vi "AnalogControl.vi"(0 "controller":refnum<k24>, 1 "analog input":i32, 2 "offset value":dbl, 3 "speed value":dbl, 5 "axis name":string, 7 "on/off":i32(ring) items=["Off", "On"], 9 "taskId":i32(ring) items=["TLibrary", "T01", "T02", "T03", "T04", "T05", "T06", "T07", "T08", "T09", "T10", "T11", "T12", "T13", "T14", "T15", "T16", "T17", "T18", "T19", "T20", "T21", "T22", "T23", "T24", "T25", "T26", "T27", "T28", "T29", "T30", "T31"], 11 "error in (no error)":errorcluster, 12 "scale factor":dbl=1.0, 13 "return immediately":bool) -> (4 "controller out":refnum<k24>, 15 "error out":errorcluster)   [LabVIEW 2020, in "Aerotech.lvlib"]
uses:
  Aerotech.lvlib
  C:/Users/HEP/Documents/GitHub/UCSB-Gantry-HEP/Drivers/Aerotech A3200/Bin/Aerotech.A3200.LabVIEW.dll
  UCSB-Gantry-HEP/Drivers/Aerotech A3200/Bin/Aerotech.A3200.LabVIEW.dll
  C:/Program Files (x86)/Aerotech/A3200/LabVIEW/2010/Bin/Aerotech.A3200.dll
  Program Files (x86)/Aerotech/A3200/LabVIEW/2010/Bin/Aerotech.A3200.dll
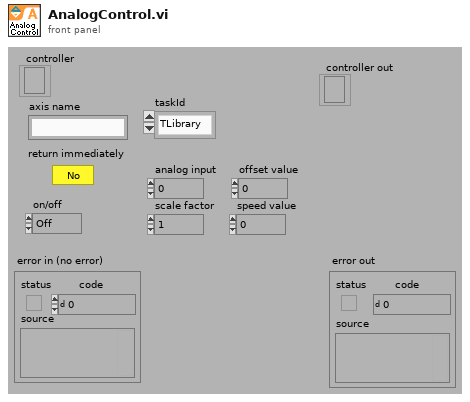
[diagram p1: front panel]
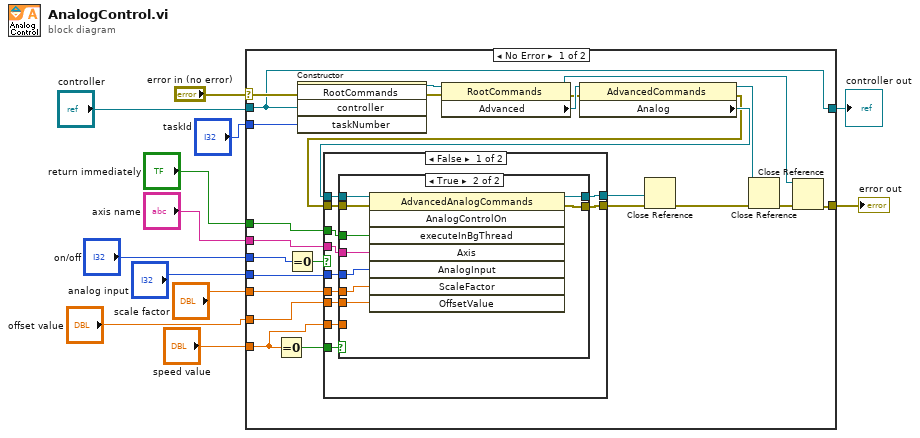
[diagram p0: block diagram]
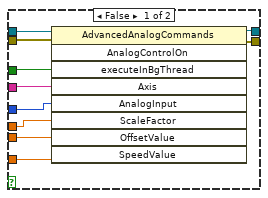
[diagram p2: hidden frame]
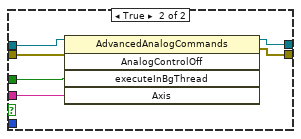
[diagram p3: hidden frame]
diagram:
  n1 = case shown="No Error" "error in (no error)" {
    selector: "error in (no error)" -> [w18 w75]
    tunnel: [w31 w75] -> w11
    tunnel: "controller" -> [w16 w74]
    tunnel: "return immediately" -> [w35 _]
    tunnel: "axis name" -> [w34 _]
    tunnel: "on/off" -> [w21 _]
    tunnel: [w16 w74] -> w1
    tunnel: "analog input" -> [w26 _]
    tunnel: "scale factor" -> [w25 _]
    tunnel: "offset value" -> [w24 _]
    tunnel: "speed value" -> [w22 _]
    tunnel: "taskId" -> [w13 _]
    frame No Error {
      n2 = Equal To 0?(x=w22) -> (x = 0?=w23:bool)
      n3 = Equal To 0?(x=w21) -> (x = 0?=w20:bool)
      n4 = constructor class="RootCommands"(error in=w18, "controller"=w16, "taskNumber"=w13) -> (reference out=w19:refnum<k24>, error out=w17:errorcluster)  [unwired: 2 in, 3 out]
      n5 = property class="RootCommands"(reference=w19, error in=w17) -> (reference out=w28:refnum<k24>, error out=w14:errorcluster, "Advanced"=w15:refnum<k24>)
      n6 = property class="AdvancedCommands"(reference=w15, error in=w14) -> (reference out=w29:refnum<k24>, error out=w36:errorcluster, "Analog"=w37:refnum<k24>)
      n7 = case shown="False" w20 {
        tunnel: w37 -> [w48 w72]
        tunnel: w36 -> [w47 w73]
        tunnel: w35 -> [w46 w71]
        tunnel: w34 -> [w45 w70]
        tunnel: [w44 w68] -> w33
        tunnel: [w43 w69] -> w32
        tunnel: w26 -> [w42 _]
        tunnel: w25 -> [w41 _]
        tunnel: w24 -> [w40 _]
        tunnel: w23 -> [w39 _]
        tunnel: w22 -> [w38 _]
        frame False {
          n8 = case shown="True" w39 {
            tunnel: w48 -> [w58 w67]
            tunnel: w47 -> [w57 w66]
            tunnel: w46 -> [w56 w65]
            tunnel: w45 -> [w55 w64]
            tunnel: [w54 w63] -> w44
            tunnel: [w53 w62] -> w43
            tunnel: w42 -> [w49 w61]
            tunnel: w41 -> [w50 w60]
            tunnel: w40 -> [w51 w59]
            tunnel: w38 -> [w52 _]
            frame False {
              n9 = invoke class="AdvancedAnalogCommands" method="AnalogControlOn"(reference=w58, error in=w57, "executeInBgThread"=w56, "Axis"=w55, "AnalogInput"=w49, "ScaleFactor"=w50, "OffsetValue"=w51, "SpeedValue"=w52) -> (reference out=w53:refnum<k24>, error out=w54:errorcluster)  [unwired: 1 in, 7 out]
            }
            frame True {
              n10 = invoke class="AdvancedAnalogCommands" method="AnalogControlOn"(reference=w67, error in=w66, "executeInBgThread"=w65, "Axis"=w64, "AnalogInput"=w61, "ScaleFactor"=w60, "OffsetValue"=w59) -> (reference out=w62:refnum<k24>, error out=w63:errorcluster)  [unwired: 1 in, 6 out]
            }
          }
        }
        frame True {
          n11 = invoke class="AdvancedAnalogCommands" method="AnalogControlOff"(reference=w72, error in=w73, "executeInBgThread"=w71, "Axis"=w70) -> (reference out=w69:refnum<k24>, error out=w68:errorcluster)  [unwired: 1 in, 3 out]
        }
      }
      n12 = Close Reference(reference=w32, error in (no error)=w33) -> (error out=w27:errorcluster)
      n13 = Close Reference(reference=w29, error in (no error)=w27) -> (error out=w30:errorcluster)
      n14 = Close Reference(reference=w28, error in (no error)=w30) -> (error out=w31:errorcluster)
    }
    frame Error {
    }
  }
  "error out" <- w11
  "controller out" <- w1
